vi "xeva-cooling.vi"(3 "error in (no error)":errorcluster, 4 "xeva-cool-on":bool=TRUE, 5 "xeva-camref":T1) -> (0 "error out":errorcluster, 1 "xeva-cooling":bool)   [LabVIEW 2017]
uses:
  <vilib>/Xenics Infrared Solutions/Xeneth LabVIEW API/VIs/Controls/Camara.ctl
  <vilib>/Xenics Infrared Solutions/Xeneth LabVIEW API/VIs/Property/XC Set Property Value L.vi
  <vilib>/Xenics Infrared Solutions/Xeneth LabVIEW API/Xeneth.lvlib
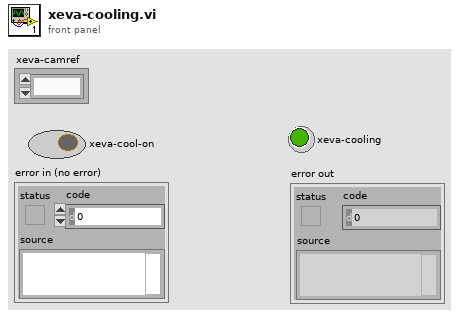
[diagram p1: front panel]
types:
  T1 = typedef "Xeneth.lvlib/Camara.ctl" = refnum<k1>
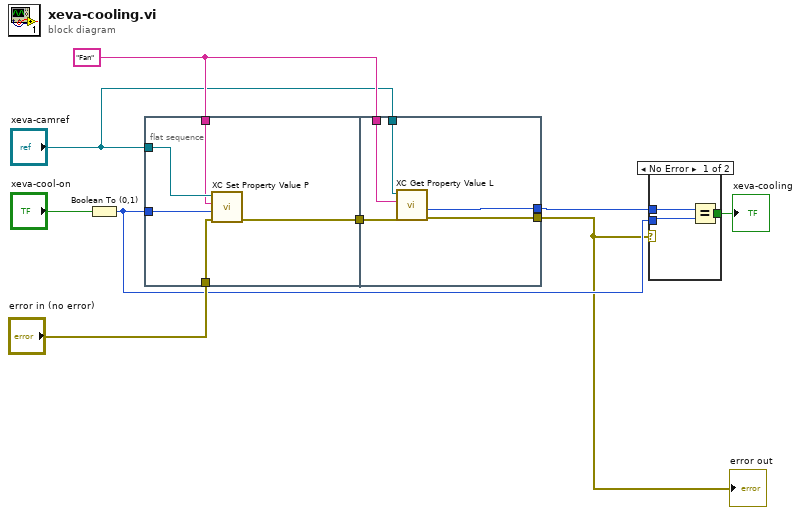
[diagram p0: block diagram]
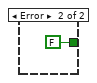
[diagram p2: hidden frame]
diagram:
  w4 = "Fan" ("pPrp")
  n1 = Boolean To (0,1)(Boolean="xeva-cool-on") -> (0, 1=w7:i16)
  n2 = flat-sequence {
    tunnel: "xeva-camref" -> [w14]
    tunnel: "error in (no error)" -> [w13]
    tunnel: w4 -> [w11]
    tunnel: w7 -> [w10]
    tunnel: [w12] -> w6
    tunnel: w6 -> [w17]
    tunnel: [w19] -> w2
    tunnel: [w18] -> w5
    tunnel: w4 -> [w16]
    tunnel: "xeva-camref" -> [w15]
    frame #0 {
      n3 = call-poly <vilib>:"XC Set Property Value P.vi"("error in (no error)"=w13, "lValue"=w10, "pPrp"=w11, "Cam Ref"=w14) -> ("error out"=w12:errorcluster)  [unwired: 6 in, 1 out]
    }
    frame #1 {
      n4 = call <vilib>:"XC Get Property Value L.vi"("error in (no error)"=w17, "pPrp"=w16, "Cam Ref"=w15) -> ("error out"=w19:errorcluster, "pValue out"=w18:i32)  [unwired: 6 in, 1 out]
    }
  }
  n5 = case shown="No Error" w2 {
    tunnel: [w22 FALSE] -> w8
    tunnel: w7 -> [w21 _]
    tunnel: w5 -> [w20 _]
    frame No Error {
      n6 = Equal?(x=w20, y=w21) -> (x = y?=w22:bool)
    }
    frame Error {
    }
  }
  "xeva-cooling" <- w8
  "error out" <- w2
